vi "PID Mindstorms.vi"() -> ()   [LabVIEW 2010]
uses:
  <vilib>/NXT/Subs/MotorOutput.ctl
  <vilib>/NXT/Dual Mode Library/Motors/Rotation.vi
  <vilib>/NXT/Dual Mode Library/Motors/MotorOn.vi
panel:
  in  "Setpoint":dbl=9.0
  out "Output":dbl
  in  "D":dbl=1.0
  in  "I":dbl
  in  "P":dbl=1.0
  in  "dt":u32=200
  out "Waveform Chart":cluster{dbl, dbl, i32, i32}(graph)
  in  "Power":i32=75
  in  "stop":bool
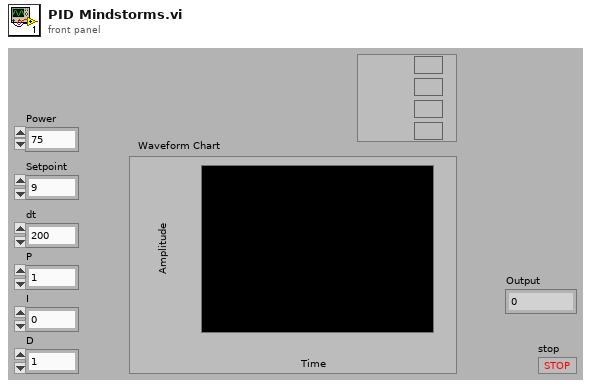
[diagram p1: front panel]
types:
  T1 = typedef "MotorOutput.ctl" = u8
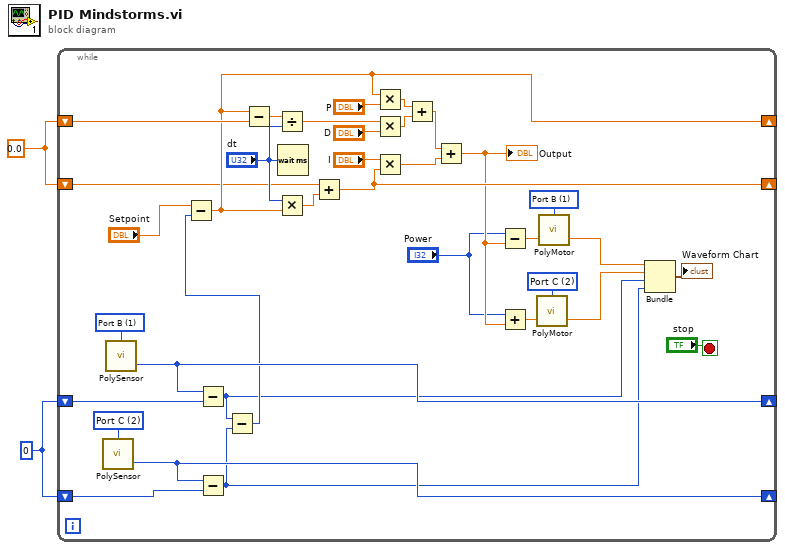
[diagram p0: block diagram]
diagram:
  w1 = 0 ("Angle of Rotation")
  w2 = 0.0
  n1 = while {
    shift-right: [w25] -> _
    shift-left: w2 -> [w32]
    shift-right: [w24] -> _
    shift-left: w2 -> [w22]
    shift-right: [w10] -> _
    shift-left: w1 -> [w9]
    shift-right: [w8] -> _
    shift-left: w1 -> [w7]
    stop <- "stop" stop-if-true
    w11 = u8 2 items=["Port A", "Port B", "Port C"] ("Port (Port A)")
    w12 = u8 1 items=["Port A", "Port B", "Port C"] ("Port (Port A)")
    w33 = T1 2 items=["Port A"=0, "Port B"=1, "Port C"=2, "Ports A & B"=4, "Ports A & C"=5, "Ports B & C"=6, "All Ports"=3] ("Output Port (All Ports)")
    w34 = T1 1 items=["Port A"=0, "Port B"=1, "Port C"=2, "Ports A & B"=4, "Ports A & C"=5, "Ports B & C"=6, "All Ports"=3] ("Output Port (All Ports)")
    n2 = call-poly <vilib>:"PolySensor.vi"("Port (Port A)"=w11) -> ("Angle of Rotation"=w8:i32)  [unwired: 2 in, 1 out]
    n3 = call-poly <vilib>:"PolySensor.vi"("Port (Port A)"=w12) -> ("Angle of Rotation"=w10:i32)  [unwired: 2 in, 1 out]
    n4 = Subtract(x=w10, y=w9) -> (x-y=w5:i32)
    n5 = Subtract(x=w8, y=w7) -> (x-y=w4:i32)
    n6 = Subtract(x=w5, y=w4) -> (x-y=w6:i32)
    n7 = Subtract(x="Setpoint", y=w6) -> (x-y=w25:dbl)
    n8 = Subtract(x=w25, y=w32) -> (x-y=w31:dbl)
    n9 = Divide(x=w31, y="dt") -> (x/y=w23:dbl)
    n10 = Multiply(x="dt", y=w25) -> (x*y=w21:dbl)
    n11 = Wait (ms)(milliseconds to wait="dt") -> ()  [unwired: 1 out]
    n12 = Add(x=w22, y=w21) -> (x+y=w24:dbl)
    n13 = Multiply(x=w25, y="P") -> (x*y=w29:dbl)
    n14 = Multiply(x=w23, y="D") -> (x*y=w28:dbl)
    n15 = Multiply(x="I", y=w24) -> (x*y=w26:dbl)
    n16 = Add(x=w29, y=w28) -> (x+y=w27:dbl)
    n17 = Add(x=w27, y=w26) -> (x+y=w16:dbl)
    "Output" <- w16
    n18 = Subtract(x="Power", y=w16) -> (x-y=w14:dbl)
    n19 = Add(x="Power", y=w16) -> (x+y=w13:dbl)
    n20 = call-poly <vilib>:"PolyMotor.vi"("Power (75)"=w13, "Output Port (All Ports)"=w33) -> ()  [unwired: 2 in, 1 out]
    n21 = call-poly <vilib>:"PolyMotor.vi"("Power (75)"=w14, "Output Port (All Ports)"=w34) -> ()  [unwired: 2 in, 1 out]
    n22 = Bundle(w14, w13, w5, w4) -> (→"Waveform Chart":cluster{dbl, dbl, i32, i32})  [unwired: 1 in]
  }
